vi "cRIO Temp Monitor.vi"() -> ()   [LabVIEW 2016]
uses:
  <vilib>/TagLibrary/Write (Double).vi
  <vilib>/TagLibrary/Read (Double).vi
  <vilib>/TagLibrary/Create Tag (Double).vi
  <vilib>/Waveform/WDTOps.llb/WDT Number of Waveform Samples DBL.vi
  <vilib>/nisyscfg/nisyscfg.lvlib
  <vilib>/NI_Real-Time Target Support.lvlib
  <vilib>/TagLibrary/TagLibrary.lvlib
  <resource>/objmgr/niTag.rc
  <resource>/objmgr/nisysapi.rc
panel:
  out "Buffer":waveform(dbl)(graph)
  out "Send File":bool
  out "Files Sent":dbl
  out "Buffered":i32
  out "AI3":dbl
  out "AI0":dbl
  out "AI2":dbl
  out "AI1":dbl
  out "Free Physical Memory":dbl
  out "Disk Free":dbl
  in  "stop":bool
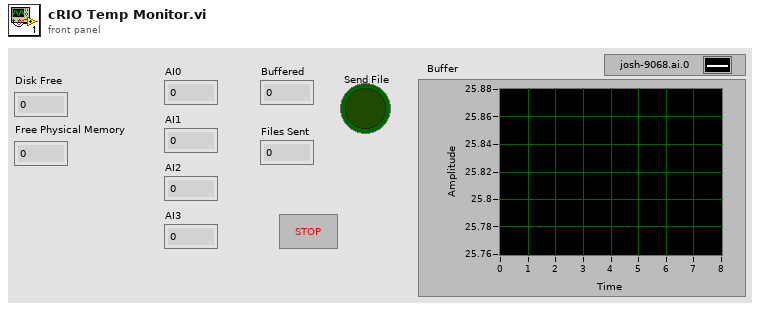
[diagram p1: front panel]
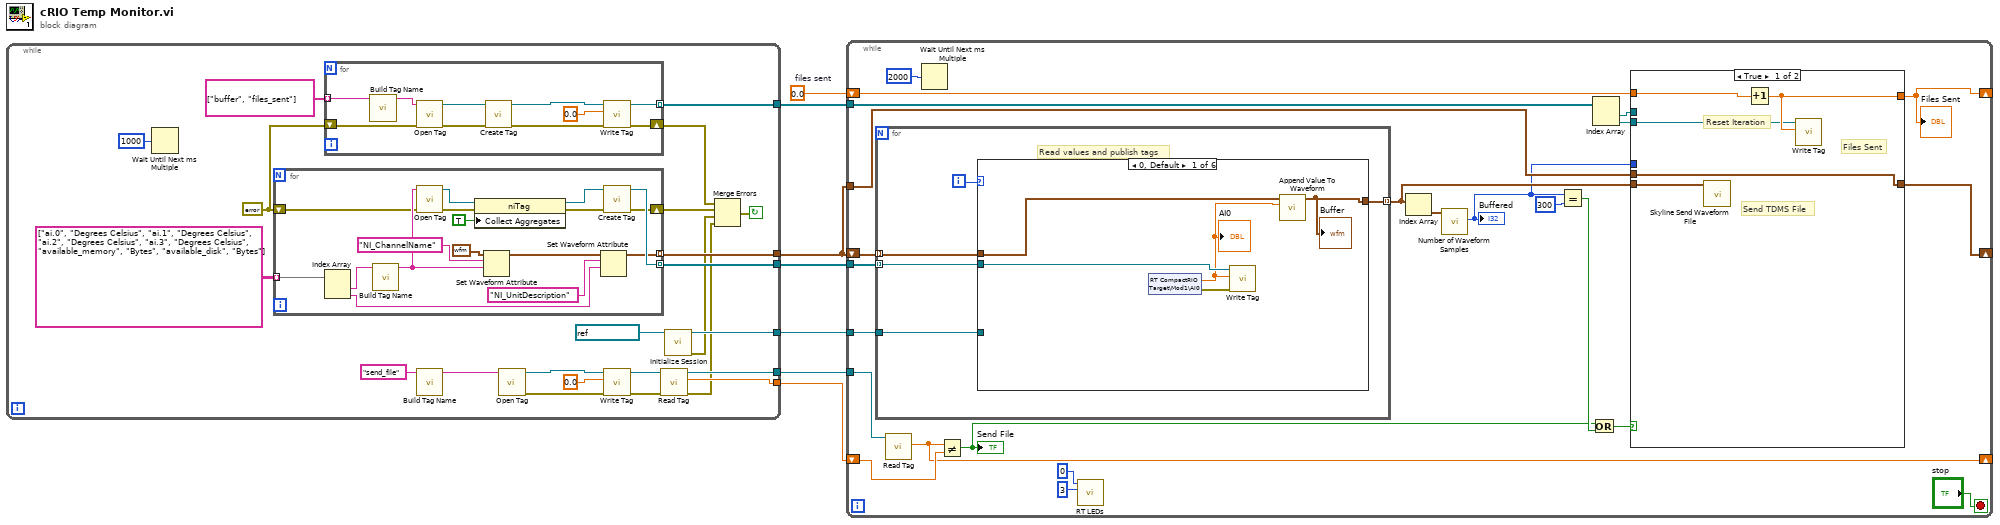
[diagram p0: block diagram]
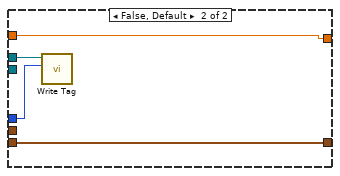
[diagram p2: hidden frame]
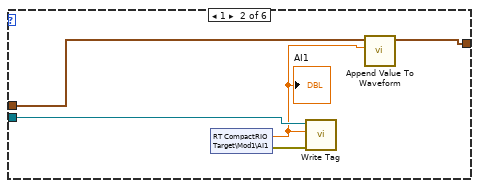
[diagram p3: hidden frame]
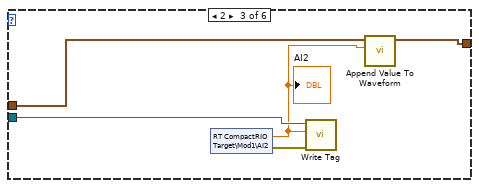
[diagram p4: hidden frame]
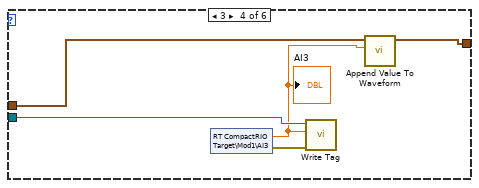
[diagram p5: hidden frame]
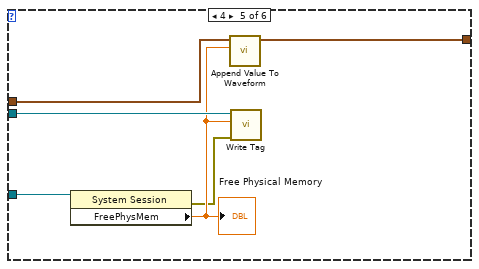
[diagram p6: hidden frame]
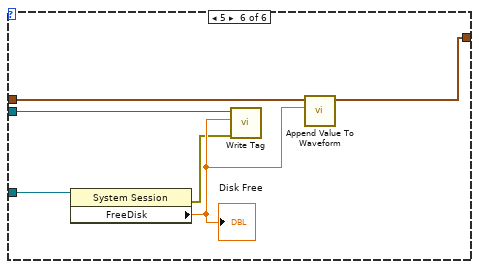
[diagram p7: hidden frame]
diagram:
  w1 = 0.0  # files sent
  n1 = while {
    tunnel: [w29] -> w7
    tunnel: [w27] -> w6
    tunnel: [w26] -> w5
    tunnel: [w24] -> w4
    tunnel: [w23] -> w3
    tunnel: [w20] -> w2
    stop <- w9 continue-if-true
    w13 = errorcluster {"status"=FALSE, "code"=0, "source"=""} ("error out")
    n2 = Wait Until Next ms Multiple(millisecond multiple=u32 1000) -> ()  [unwired: 1 out]
    n3 = for {
      tunnel: string[][] [["ai.0", "Degrees Celsius"], ["ai.1", "Degrees Celsius"], ["ai.2", "Degrees Celsius"], ["ai.3", "Degrees Celsius"], ["available_memory", "Bytes"], ["available_disk", "Bytes"]] -> [w46] mode=indexing
      tunnel: [w52] -> w29 mode=indexing
      tunnel: [w43] -> w27 mode=indexing
      shift-right: [w42] -> w12
      shift-left: w13 -> [w41]
      n4 = Index Array(array=w46) -> (element #1=w44:string, element #2=w45:string)  [unwired: 2 in]
      n5 = call "Build Tag Name.vi"("Tag"=w44) -> ("System Tag"=w47:string)  [unwired: 10 in]
      n6 = call <vilib>:"Open Tag.vi"("error in (no error)"=w41, "tag path"=w47) -> ("error out"=w54:errorcluster, "tag reference out"=w57:refnum<k21>)  [unwired: 8 in]
      n7 = property class="niTag"(reference=w57, error in=w54, "Collect Aggregates"=TRUE) -> (reference out=w56:refnum<k21>, error out=w55:errorcluster)
      n8 = Set Waveform Attribute(5:w47, 6:"NI_ChannelName" ("name"), 7:waveform(dbl) {"t0"=timestamp(0 s since 1904-01-01), "dt"=1.0, "Y"=[]} ("waveform")) -> (3:w49:waveform(dbl))  [unwired: 1 in, 2 out]
      n9 = Set Waveform Attribute(5:w45, 6:"NI_UnitDescription" ("name"), 7:w49) -> (3:w43:waveform(dbl))  [unwired: 1 in, 2 out]
      n10 = call-poly <vilib>:"Create Tag.vi"("error in (no error)"=w55, "tag reference in"=w56) -> ("error out"=w42:errorcluster, "tag reference out"=w52:refnum<k21>)  [unwired: 8 in]
    }
    n11 = for {
      tunnel: [w37] -> w26 mode=indexing
      tunnel: string[] ["buffer", "files_sent"] -> [w35] mode=indexing
      shift-right: [w32] -> w14
      shift-left: w13 -> [w31]
      n12 = call "Build Tag Name.vi"("Tag"=w35) -> ("System Tag"=w38:string)  [unwired: 10 in]
      n13 = call <vilib>:"Open Tag.vi"("error in (no error)"=w31, "tag path"=w38) -> ("error out"=w33:errorcluster, "tag reference out"=w34:refnum<k21>)  [unwired: 8 in]
      n14 = call-poly <vilib>:"Create Tag.vi"("error in (no error)"=w33, "tag reference in"=w34) -> ("error out"=w40:errorcluster, "tag reference out"=w39:refnum<k21>)  [unwired: 8 in]
      n15 = call-poly <vilib>:"Write Tag.vi"("error in (no error)"=w40, "double"=0.0 ("y"), "tag reference in"=w39) -> ("error out"=w32:errorcluster, "tag reference out"=w37:refnum<k21>)  [unwired: 7 in]
    }
    n16 = call "Build Tag Name.vi"("Tag"="send_file") -> ("System Tag"=w22:string)  [unwired: 10 in]
    n17 = call <vilib>:"Open Tag.vi"("tag path"=w22) -> ("error out"=w18:errorcluster, "tag reference out"=w19:refnum<k21>)  [unwired: 9 in]
    n18 = call-poly <vilib>:"Write Tag.vi"("error in (no error)"=w18, "double"=0.0 ("y"), "tag reference in"=w19) -> ("error out"=w15:errorcluster, "tag reference out"=w16:refnum<k21>)  [unwired: 7 in]
    n19 = call-poly <vilib>:"Read Tag.vi"("error in (no error)"=w15, "tag reference in"=w16) -> ("error out"=w10:errorcluster, "double"=w24:dbl, "tag reference out"=w23:refnum<k21>)  [unwired: 5 in, 2 out]
    n20 = call <vilib>:"Initialize Session.vi"("Target (localhost)"=refnum<k21> "localhost") -> ("error out"=w11:errorcluster, "Session out"=w20:refnum<k21>)  [unwired: 9 in]
    n21 = Merge Errors(w14, w12, w11, w10) -> (w9:errorcluster)
  }
  n22 = while {
    tunnel: w7 -> [w77]
    shift-right: [w75] -> _
    shift-left: w6 -> [w76]
    tunnel: w6 -> [w74]
    tunnel: w5 -> [w68]
    shift-right: [w69] -> _
    shift-left: w1 -> [w70]
    tunnel: w3 -> [w64]
    shift-right: [w63] -> _
    shift-left: w4 -> [w65]
    tunnel: w2 -> [w61]
    stop <- "stop" stop-if-true
    n23 = for {
      tunnel: w77 -> [w94] mode=indexing
      tunnel: w76 -> [w93] mode=indexing
      tunnel: [w92] -> w60 mode=indexing
      tunnel: w61 -> [w91]
      i -> [w95]
      # "Read values and publish tags"
      n24 = case shown="0, Default" w95 {
        tunnel: w94 -> [w99 w104 w109 w114 w121 w127]
        tunnel: w93 -> [w98 w103 w108 w113 w120 w126]
        tunnel: [w96 w101 w107 w112 w118 w125] -> w92
        tunnel: w91 -> [_ _ _ _ w117 w123]
        frame 0, Default {
          n25 = shared-variable "RT CompactRIO Target\\Mod1\\AI0"() -> (w97:dbl, error out=w100:errorcluster)  [unwired: 1 in]
          "AI0" <- w97
          n26 = call-poly <vilib>:"Write Tag.vi"("error in (no error)"=w100, "double"=w97, "tag reference in"=w99) -> ()  [unwired: 7 in, 2 out]
          n27 = call "Append Value To Waveform.vi"("Numeric"=w97, "waveform in"=w98) -> ("waveform out"=w96:waveform(dbl))  [unwired: 9 in]
          "Buffer" <- w96
        }
        frame 1 {
          n28 = shared-variable "RT CompactRIO Target\\Mod1\\AI1"() -> (w102:dbl, error out=w105:errorcluster)  [unwired: 1 in]
          "AI1" <- w102
          n29 = call-poly <vilib>:"Write Tag.vi"("error in (no error)"=w105, "double"=w102, "tag reference in"=w104) -> ()  [unwired: 7 in, 2 out]
          n30 = call "Append Value To Waveform.vi"("Numeric"=w102, "waveform in"=w103) -> ("waveform out"=w101:waveform(dbl))  [unwired: 9 in]
        }
        frame 2 {
          n31 = shared-variable "RT CompactRIO Target\\Mod1\\AI2"() -> (w106:dbl, error out=w110:errorcluster)  [unwired: 1 in]
          "AI2" <- w106
          n32 = call-poly <vilib>:"Write Tag.vi"("error in (no error)"=w110, "double"=w106, "tag reference in"=w109) -> ()  [unwired: 7 in, 2 out]
          n33 = call "Append Value To Waveform.vi"("Numeric"=w106, "waveform in"=w108) -> ("waveform out"=w107:waveform(dbl))  [unwired: 9 in]
        }
        frame 3 {
          n34 = shared-variable "RT CompactRIO Target\\Mod1\\AI3"() -> (w111:dbl, error out=w115:errorcluster)  [unwired: 1 in]
          "AI3" <- w111
          n35 = call-poly <vilib>:"Write Tag.vi"("error in (no error)"=w115, "double"=w111, "tag reference in"=w114) -> ()  [unwired: 7 in, 2 out]
          n36 = call "Append Value To Waveform.vi"("Numeric"=w111, "waveform in"=w113) -> ("waveform out"=w112:waveform(dbl))  [unwired: 9 in]
        }
        frame 4 {
          n37 = property class="System Session"(reference=w117) -> (error out=w116:errorcluster, "FreePhysMem"=w119:dbl)  [unwired: 1 in, 1 out]
          "Free Physical Memory" <- w119
          n38 = call "Append Value To Waveform.vi"("Numeric"=w119, "waveform in"=w120) -> ("waveform out"=w118:waveform(dbl))  [unwired: 9 in]
          n39 = call-poly <vilib>:"Write Tag.vi"("error in (no error)"=w116, "double"=w119, "tag reference in"=w121) -> ()  [unwired: 7 in, 2 out]
        }
        frame 5 {
          n40 = property class="System Session"(reference=w123) -> (error out=w122:errorcluster, "FreeDisk"=w124:dbl)  [unwired: 1 in, 1 out]
          "Disk Free" <- w124
          n41 = call-poly <vilib>:"Write Tag.vi"("error in (no error)"=w122, "double"=w124, "tag reference in"=w127) -> ()  [unwired: 7 in, 2 out]
          n42 = call "Append Value To Waveform.vi"("Numeric"=w124, "waveform in"=w126) -> ("waveform out"=w125:waveform(dbl))  [unwired: 9 in]
        }
      }
    }
    n43 = call-poly <vilib>:"Read Tag.vi"("tag reference in"=w64) -> ("double"=w63:dbl)  [unwired: 6 in, 4 out]
    n44 = Wait Until Next ms Multiple(millisecond multiple=u32 2000) -> ()  [unwired: 1 out]
    n45 = Not Equal?(x=w63, y=w65) -> (x != y?=w62:bool)
    "Send File" <- w62
    n46 = call <vilib>:"RT LEDs.vi"("State"=3, "LED Num"=0) -> ()  [unwired: 4 in, 2 out]
    n47 = Index Array(array=w60) -> (element=w59:waveform(dbl))  [unwired: 1 in]
    n48 = call-poly <vilib>:"Number of Waveform Samples.vi"("waveform in"=w59) -> ("number of samples"=w58:i32)  [unwired: 8 in, 2 out]
    "Buffered" <- w58
    n49 = Equal?(x=w58, y=300) -> (x = y?=w73:bool)
    n50 = Or(x=w62, y=w73) -> (x .or. y?=w72:bool)
    n51 = Index Array(array=w68) -> (element #1=w67:refnum<k21>, element #2=w66:refnum<k21>)  [unwired: 2 in]
    n52 = case shown="True" w72 {
      tunnel: w60 -> [w86 w89]
      tunnel: [w85 w89] -> w75
      tunnel: w74 -> [w85 _]
      tunnel: w70 -> [w84 w90]
      tunnel: [w83 w90] -> w69
      tunnel: w58 -> [_ w88]
      tunnel: w67 -> [_ w87]
      tunnel: w66 -> [w82 _]
      frame True {
        # "Files Sent"
        # "Reset Iteration"
        # "Send TDMS File"
        n53 = call "Skyline Send Waveform File.vi"("data in"=w86) -> ()  [unwired: 8 in, 3 out]
        n54 = Increment(x=w84) -> (x+1=w83:dbl)
        n55 = call-poly <vilib>:"Write Tag.vi"("double"=w83, "tag reference in"=w82) -> ()  [unwired: 8 in, 2 out]
      }
      frame False, Default {
        n56 = call-poly <vilib>:"Write Tag.vi"("double"=w88, "tag reference in"=w87) -> ()  [unwired: 8 in, 2 out]
      }
    }
    "Files Sent" <- w69
  }
